vi "AAL_TimeSeries_ErrorCode.vi"() -> ()   [LabVIEW 2012, in "NI_AALPro.lvlib"]
uses:
  NI_AALPro.lvlib
panel:
  in  "DtGTZeroErr":i32=-20016
  in  "time not in ascending order":i32=-20077
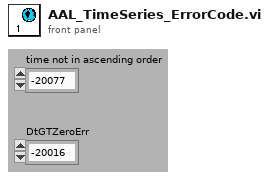
[diagram p1: front panel]
diagram:
